vi "Read Gate Delay Position (Scan).vi"(8 "error in (no error)":errorcluster, 10 "Gate (A)":T1, 11 "VISA resource name":refnum<visa-resource-name>) -> (0 "error out":errorcluster, 1 "Gate Delay Position":dbl format="%#_4e", 3 "VISA resource name out":refnum<visa-resource-name>)   [LabVIEW 2013, in "SRS SR400.lvlib"]
doc: "<B>GZ i</B>\n\nThe GZ command returns the gate delay position during a scan. i = 0 or 1 designates A gate or B gate and is required. If gate i is in the SCAN mode, its current delay position during a scan is read. If the counters are in reset or the gate is not in the SCAN mode, the GZ command returns the starting delay position (same as GD command). The GZ command is a read only command."
uses:
  <instrlib>/SRS SR400/SRS SR400.lvlib
  <instrlib>/SRS SR400/Public/Typedefs/Gate.ctl
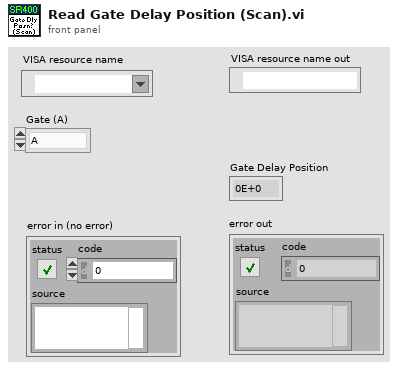
[diagram p1: front panel]
types:
  T1 = typedef "SRS SR400.lvlib/Gate.ctl" = enum16{"A", "B"}
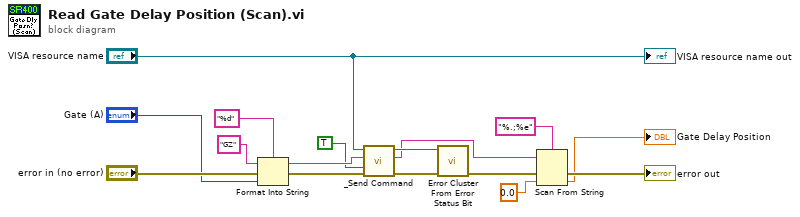
[diagram p0: block diagram]
diagram:
  n1 = Format Into String(format string="%d", initial string="GZ" ("command"), error in="error in (no error)", "Gate (A)") -> (resulting string=w9:string, error out=w8:errorcluster)
  n2 = call <instrlib>:"_Send Command.vi"("error in (no error)"=w8, "Read Value? (F)"=TRUE, "Command"=w9, "VISA resource name"="VISA resource name") -> ("error out"=w3:errorcluster, "Response"=w1:string, "VISA resource name out"=w4:refnum<visa-resource-name>)  [unwired: 5 out]
  n3 = call <instrlib>:"Error Cluster From Error Status Bit.vi"("error in (no error)"=w3, "VISA resource name"=w4) -> ("error out"=w2:errorcluster)  [unwired: 8 in, 1 out]
  n4 = Scan From String(format string="%.;%e", input string=w1, error in=w2, default 1=0.0 ("default value 1")) -> (error out=→"error out":errorcluster, output 1=→"Gate Delay Position":dbl)  [unwired: 1 in, 2 out]
  "VISA resource name out" <- "VISA resource name"
